vi "MaxAreaIndex.vi"(11 "Region Reports":T1(array[cluster]) {"Mean Value" format="%.2f"; "%" format="%.2f"; "Area (calibrated)" format="%.2f"; "Maximal Value" format="%.2f"; "Minimal Value" format="%.2f"; "Standard Variation" format="%.2f"}) -> (3 "Index":i32)   [LabVIEW 2016]
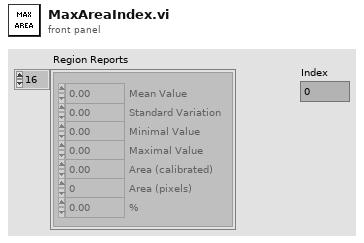
[diagram p1: front panel]
types:
  T1 = cluster{"Mean Value":sgl, "Standard Variation":sgl, "Minimal Value":sgl, "Maximal Value":sgl, "Area (calibrated)":sgl, "Area (pixels)":i32, "%":sgl}[]
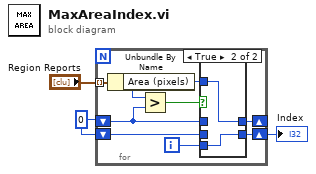
[diagram p0: block diagram]
diagram:
  w3 = 0
  n1 = for {
    tunnel: "Region Reports" -> [w11] mode=indexing
    shift-right: [w8] -> _
    shift-left: w3 -> [w7]
    shift-right: [w5] -> w1
    shift-left: w3 -> [w6]
    i -> [w4]
    n2 = Unbundle By Name(w11) -> ("Area (pixels)"=w9:i32)
    n3 = Greater?(x=w9, y=w7) -> (0:w10:bool)
    n4 = case shown="True" w10 {
      tunnel: w9 -> [_ w15]
      tunnel: [w13 w15] -> w8
      tunnel: w7 -> [w13 _]
      tunnel: w6 -> [w12 _]
      tunnel: [w12 w14] -> w5
      tunnel: w4 -> [_ w14]
      frame False {
      }
      frame True {
      }
    }
  }
  "Index" <- w1
